vi "Split U32.vi"(7 "LSB Length":u8=4, 11 "U32":u32 format="%x") -> (2 "LSB":u32 format="%x", 3 "MSB":u32 format="%x")   [LabVIEW 2021, in "DataTypes_CIF_U.lvlib"]
doc: "This will split a byte into two numbers each using a subset of the bits. The MSB for Ethernet is the portion of the byte that contains bit 0."
uses:
  DataTypes_CIF_U.lvlib
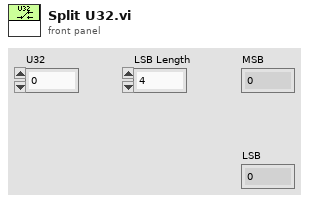
[diagram p1: front panel]
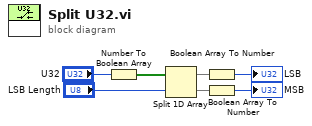
[diagram p0: block diagram]
diagram:
  n1 = Number To Boolean Array(number="U32") -> (Boolean array=w5:bool[])
  n2 = Split 1D Array(array=w5, index="LSB Length") -> (first subarray=w7:bool[], second subarray=w6:bool[])
  n3 = Boolean Array To Number(Boolean array=w7) -> (number=→"LSB":u32)
  n4 = Boolean Array To Number(Boolean array=w6) -> (number=→"MSB":u32)
